vi "AI AO.vi"() -> ()   [LabVIEW 2026]
uses:
  <vilib>/DAQmx/read.llb/DAQmx Read (Analog DBL 1Chan 1Samp).vi
  <vilib>/DAQmx/write.llb/DAQmx Write (Analog DBL 1Chan 1Samp).vi
  <vilib>/DAQmx/create/channels.llb/DAQmx Create Channel (AI-Voltage-Basic).vi
  <vilib>/DAQmx/configure/timing.llb/DAQmx Timing (Sample Clock).vi
  <vilib>/DAQmx/create/channels.llb/DAQmx Create Channel (AO-Voltage-Basic).vi
  <vilib>/DAQmx/miscellaneous.llb/DAQmx Fill In Error Info.vi
  <resource>/objmgr/daqmx.rc
panel:
  out "Input.BufSize":u32
  out "task done? AO":bool
  out "task done? AI":bool
  in  "data":dbl(slide) scale=-5.0..5.0
  out "data":dbl(slide) scale=-5.0..5.0
  in  "stop":bool
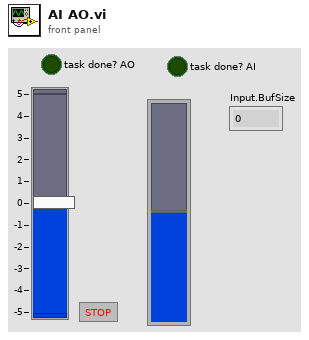
[diagram p1: front panel]
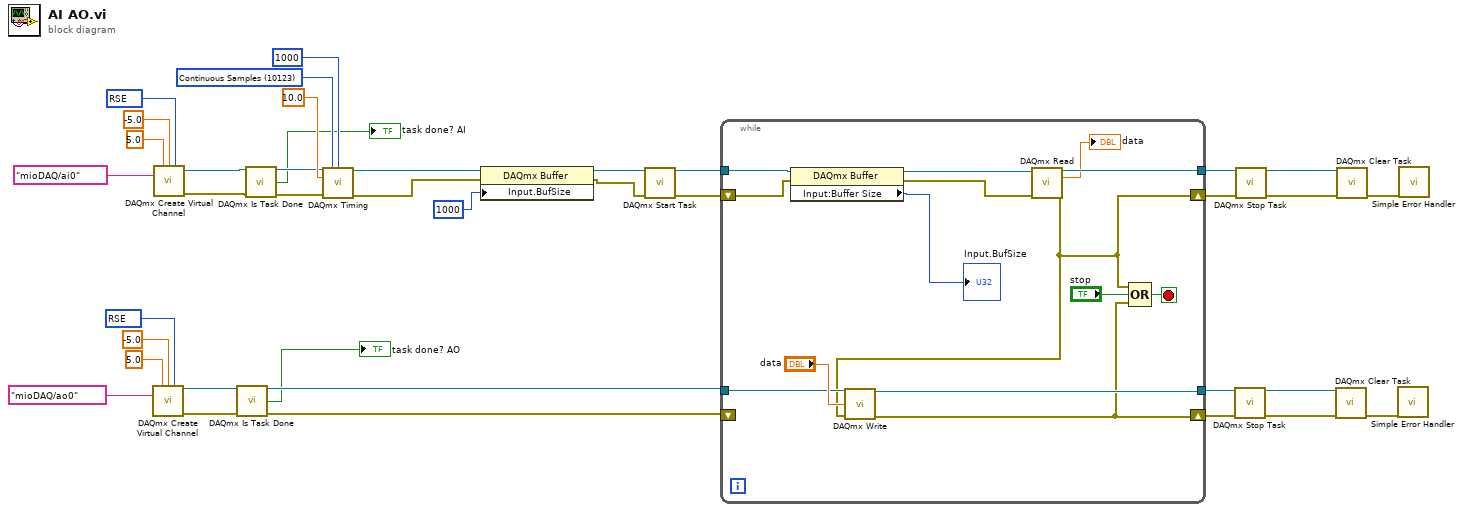
[diagram p0: block diagram]
diagram:
  w23 = 10083 items=["Default"=-1, "RSE"=10083, "NRSE"=10078, "Differential"=10106, "Pseudodifferential"=12529] ("input terminal configuration")
  w26 = 10083 items=["Default"=-1, "RSE"=10083, "NRSE"=10078, "Differential"=10106, "Pseudodifferential"=12529] ("input terminal configuration")
  w31 = 10123 items=["Finite Samples"=10178, "Continuous Samples"=10123, "Hardware Timed Single Point"=12522] ("sample mode")
  n1 = call-poly <vilib>:"DAQmx Create Virtual Channel.vi"("maximum value"=5.0, "minimum value"=-5.0, "output terminal configuration"=w23, "physical channels"=tag "mioDAQ/ao0") -> ("task out"=w8:refnum<k21>, "error out"=w19:errorcluster)  [unwired: 10 in]
  n2 = call-poly <vilib>:"DAQmx Create Virtual Channel.vi"("maximum value"=5.0, "minimum value"=-5.0, "input terminal configuration"=w26, "physical channels"=tag "mioDAQ/ai0") -> ("task out"=w14:refnum<k21>, "error out"=w13:errorcluster)  [unwired: 10 in]
  n3 = call <vilib>:"DAQmx Is Task Done.vi"("task/channels in"=w8, "error in"=w19) -> ("task out"=w7:refnum<k21>, "task done?"=→"task done? AO":bool, "error out"=w9:errorcluster)  [unwired: 11 in]
  n4 = call <vilib>:"DAQmx Is Task Done.vi"("task/channels in"=w14, "error in"=w13) -> ("task out"=w11:refnum<k21>, "task done?"=→"task done? AI":bool, "error out"=w12:errorcluster)  [unwired: 11 in]
  n5 = call-poly <vilib>:"DAQmx Timing.vi"("task/channels in"=w11, "sample mode"=w31, "samples per channel"=1000, "rate"=10.0, "error in"=w12) -> ("task out"=w5:refnum<k21>, "error out"=w4:errorcluster)  [unwired: 9 in]
  n6 = property class="DAQmx Buffer"(reference=w5, error in=w4, "Input.BufSize"=u32 1000) -> (reference out=w3:refnum<k21>, error out=w2:errorcluster)
  n7 = call <vilib>:"DAQmx Start Task.vi"("task/channels in"=w3, "error in"=w2) -> ("task out"=w33:refnum<k21>, "error out"=w34:errorcluster)  [unwired: 12 in]
  n8 = while {
    shift-right: [w39] -> w38
    shift-left: w34 -> [w43]
    tunnel: w33 -> [w44]
    tunnel: [w50] -> w32
    shift-right: [w45] -> w15
    shift-left: w9 -> [_]
    tunnel: w7 -> [w47]
    tunnel: [w46] -> w20
    stop <- w51 stop-if-true
    n9 = property class="DAQmx Buffer"(reference=w44, error in=w43) -> (reference out=w42:refnum<k21>, error out=w41:errorcluster, "Input:Buffer Size"=→"Input.BufSize":u32)
    n10 = call-poly <vilib>:"DAQmx Read.vi"("task/channels in"=w42, "error in"=w41) -> ("task out"=w50:refnum<k21>, "data"=→"data":dbl, "error out"=w39:errorcluster)  [unwired: 11 in]
    n11 = call-poly <vilib>:"DAQmx Write.vi"("task/channels in"=w47, "data"="data", "error in"=w39) -> ("task out"=w46:refnum<k21>, "error out"=w45:errorcluster)  [unwired: 10 in, 1 out]
    n12 = Compound Arithmetic op=OR(w39, "stop", w45) -> (w51:bool)
  }
  n13 = call <vilib>:"DAQmx Stop Task.vi"("task/channels in"=w20, "error in"=w15) -> ("task out"=w17:refnum<k21>, "error out"=w16:errorcluster)  [unwired: 12 in]
  n14 = call <vilib>:"DAQmx Stop Task.vi"("task/channels in"=w32, "error in"=w38) -> ("task out"=w36:refnum<k21>, "error out"=w37:errorcluster)  [unwired: 12 in]
  n15 = call <vilib>:"DAQmx Clear Task.vi"("task in"=w17, "error in"=w16) -> ("error out"=w18:errorcluster)  [unwired: 13 in]
  n16 = call <vilib>:"DAQmx Clear Task.vi"("task in"=w36, "error in"=w37) -> ("error out"=w35:errorcluster)  [unwired: 13 in]
  n17 = call <vilib>:"Simple Error Handler.vi"("error in (no error)"=w18) -> ()  [unwired: 4 in, 5 out]
  n18 = call <vilib>:"Simple Error Handler.vi"("error in (no error)"=w35) -> ()  [unwired: 4 in, 5 out]
